vi "Interpolate Object To Base.vi"(7 "Table":dbl[][](array[numeric]) format="%#.1f", 8 "Y":dbl, 9 "Z":dbl, 11 "X":dbl) -> (0 "y":dbl, 1 "z":dbl, 2 "a":dbl, 3 "x":dbl)   [LabVIEW 2013]
panel:
  out "result":dbl
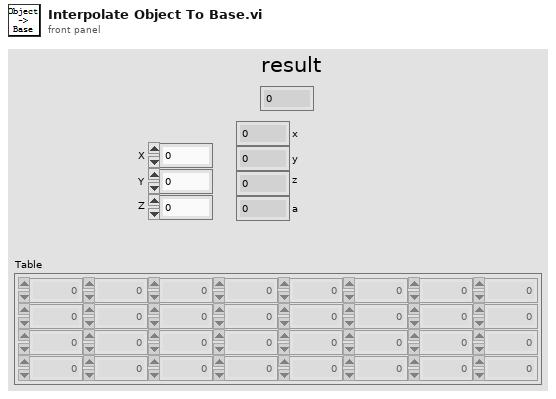
[diagram p1: front panel]
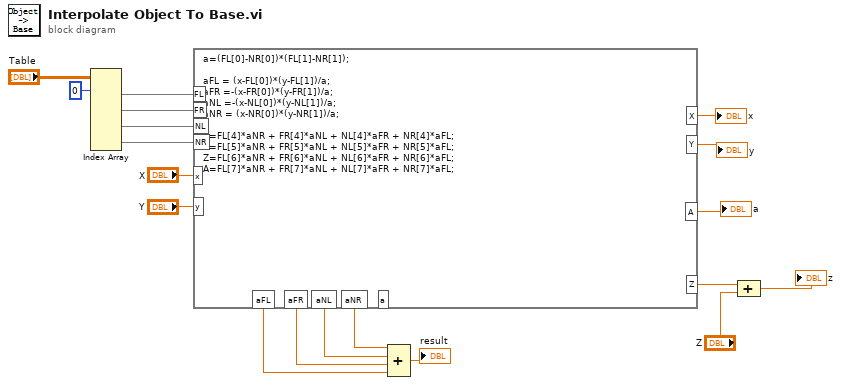
[diagram p0: block diagram]
diagram:
  n1 = Index Array(array="Table", index (row) #1=0 ("index (row)")) -> (element #1=w6:dbl[], element #2=w5:dbl[], element #3=w4:dbl[], element #4=w3:dbl[])  [unwired: 7 in]
  n2 = formula code="a=(FL[0]-NR[0])*(FL[1]-NR[1]);\n\naFL = (x-FL[0])*(y-FL[1])/a;\naFR =-(x-FR[0])*(y-FR[1])/a;\naNL =-(x-NL[0])*(y-NL[1])/a;\naNR = (x-NR[0])*(y-NR[1])/a;\n\nX=FL[4]*aNR + FR[4]*aNL + NL[4]*aFR + NR[4]*aFL;\nY=FL[5]*aNR + FR[5]*aNL + NL[5]*aFR + NR[5]*aFL;\nZ=FL[6]*aNR + FR[6]*aNL + NL[6]*aFR + NR[6]*aFL;\nA=FL[7]*aNR + FR[7]*aNL + NL[7]*aFR + NR[7]*aFL;"("x"="X", "y"="Y", "FL"=w6, "FR"=w5, "NL"=w4, "NR"=w3) -> ("aFL"=w10:dbl, "aFR"=w11:dbl, "aNL"=w12:dbl, "aNR"=w13:dbl, "X"=→"x":dbl, "Y"=→"y":dbl, "Z"=w15:dbl, "A"=→"a":dbl)  [unwired: 1 out]
  n3 = Compound Arithmetic op=ADD(w13, w12, w11, w10) -> (→"result":dbl)
  n4 = Compound Arithmetic op=ADD(w15, "Z") -> (→"z":dbl)
